vi "waitForNewWaveforms.vi"(8 "error in (no error)":errorcluster, 11 "Instrument.LockinAPI in":refnum<class "Instrument.LockinAPI.lvclass">) -> (0 "error out":errorcluster, 2 "Newest AI Waveform":waveform(dbl)[](array[waveform]), 3 "Instrument.LockinAPI out":refnum<class "Instrument.LockinAPI.lvclass">)   [LabVIEW 2019, in "Instrument.LockinAPI.lvclass"]
uses:
  Instrument.LockinAPI.lvclass
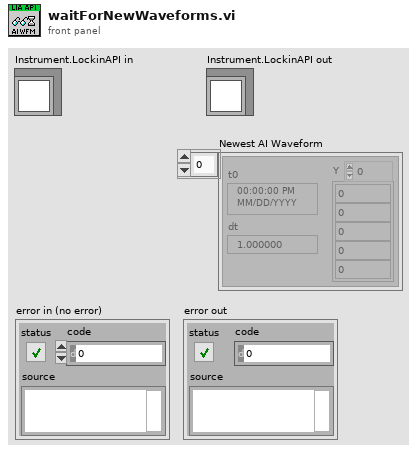
[diagram p1: front panel]
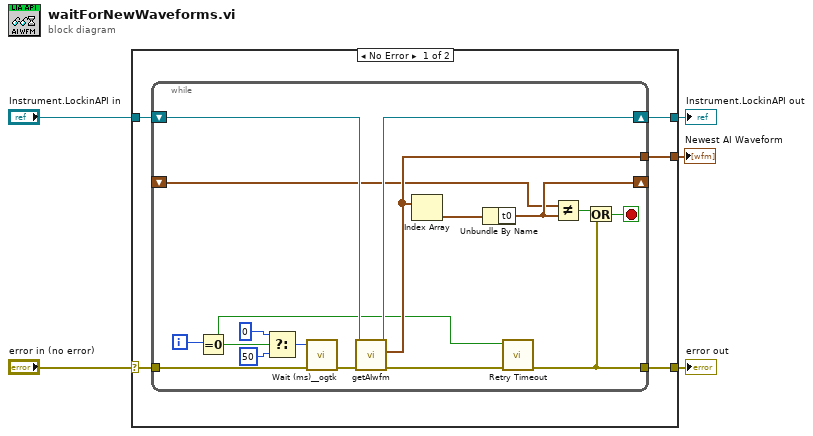
[diagram p0: block diagram]
diagram:
  n1 = case shown="No Error" "error in (no error)" {
    selector: "error in (no error)" -> [w6 w28]
    tunnel: [w10 w28] -> w5
    tunnel: [w9 _] -> w4
    tunnel: "Instrument.LockinAPI in" -> [w7 w29]
    tunnel: [w8 w29] -> w1
    frame No Error {
      n2 = while {
        shift-right: [w25] -> _
        shift-left: _ -> [w13]
        tunnel: w6 -> [w26]
        tunnel: [w16] -> w10
        tunnel: [w24] -> w9
        shift-right: [w22] -> w8
        shift-left: w7 -> [w23]
        i -> [w12]
        stop <- w20 stop-if-true
        n3 = Equal To 0?(x=w12) -> (x = 0?=w11:bool)
        n4 = Select(t=u32 0, s=w11, f=u32 50 ("milliseconds to wait")) -> (s? t:f=w17:u32)
        n5 = call <userlib>:"Wait (ms)__ogtk.vi"("error in (no error)"=w26, "milliseconds to wait"=w17) -> ("error out"=w14:errorcluster)  [unwired: 8 in, 1 out]
        n6 = call-dynamic "getAIwfm.vi"("error in (no error)"=w14, "Instrument.LockinAPI in"=w23) -> ("error out"=w15:errorcluster, "AI Waveform"=w24:waveform(dbl)[], "Instrument.LockinAPI out"=w22:refnum<class "Instrument.LockinAPI.lvclass">)  [unwired: 7 in]
        n7 = Index Array(array=w24) -> (element=w27:waveform(dbl))  [unwired: 1 in]
        n8 = Unbundle By Name(w27) -> ("t0"=w25:timestamp)
        n9 = call "Retry Timeout.vi"("error in (no error)"=w15, "reset"=w11) -> ("error out"=w16:errorcluster)  [unwired: 8 in, 1 out]
        n10 = Not Equal?(x=w13, y=w25) -> (x != y?=w21:bool)
        n11 = Or(x=w21, y=w16) -> (x .or. y?=w20:bool)
      }
    }
    frame Error {
    }
  }
  "error out" <- w5
  "Newest AI Waveform" <- w4
  "Instrument.LockinAPI out" <- w1
